vi "send interpolated data.vi"(8 "error in (no error)":errorcluster, 11 "Autofocus in":refnum<class "Autofocus.lvclass">) -> (0 "error out":errorcluster, 3 "Autofocus out":refnum<class "Autofocus.lvclass">)   [LabVIEW 2012, in "Autofocus.lvclass"]
uses:
  Autofocus.lvclass
  Autofocus.lvclass/Autofocus.ctl
  <vilib>/Distrio/Murmex/Murmex/Murmex.lvclass
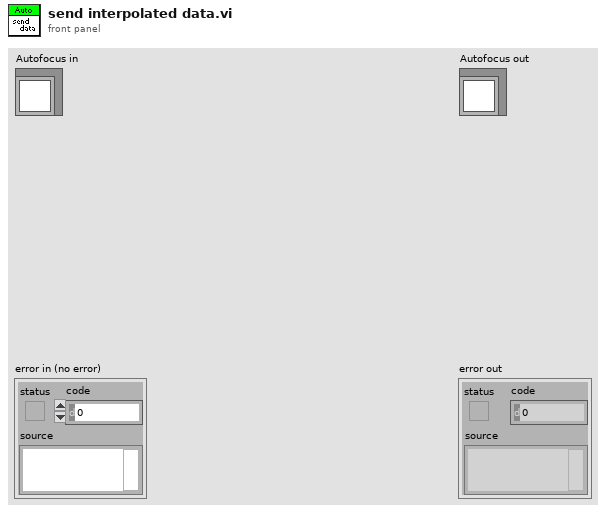
[diagram p1: front panel]
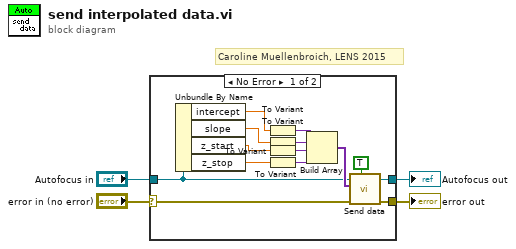
[diagram p0: block diagram]
diagram:
  # "Caroline Muellenbroich, LENS 2015"
  n1 = case shown="No Error" "error in (no error)" {
    selector: "error in (no error)" -> [w16 w20]
    tunnel: [w15 w20] -> w3
    tunnel: [w14 w19] -> w1
    tunnel: "Autofocus in" -> [w9 w19]
    frame No Error {
      n2 = Unbundle By Name(w9) -> ("intercept"=w8:dbl, "slope"=w7:dbl, "z_start"=w6:dbl[unit], "z_stop"=w5:dbl[unit])
      n3 = To Variant(anything=w8) -> (Variant=w10:variant)
      n4 = To Variant(anything=w7) -> (Variant=w11:variant)
      n5 = To Variant(anything=w6) -> (Variant=w13:variant)
      n6 = To Variant(anything=w5) -> (Variant=w12:variant)
      n7 = Build Array(w10, w11, w13, w12) -> (w17:variant[])
      n8 = call <vilib>:"Send data.vi"("is finalised data? (T)"=TRUE, "error in (no error)"=w16, "data (channels array)"=w17, "Murmex in"=w9) -> ("error out"=w15:errorcluster, "Murmex out"=w14:refnum<class "Autofocus.lvclass">)  [unwired: 6 in]
    }
    frame Error {
    }
  }
  "error out" <- w3
  "Autofocus out" <- w1
